vi "示波器主程序.vi"() -> ()   [LabVIEW 2018]
panel:
  in  "VISA资源名称":refnum<visa-resource-name>
  in  "要打开的通道":string[](array[string])
  out "波形图":u8[][](graph)
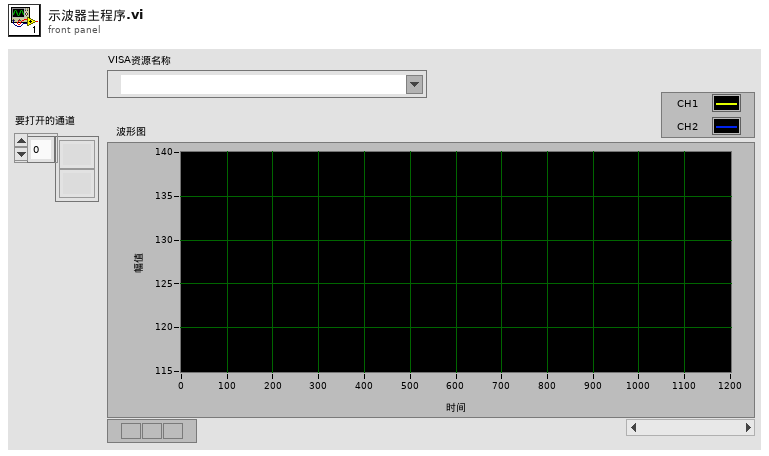
[diagram p1: front panel]
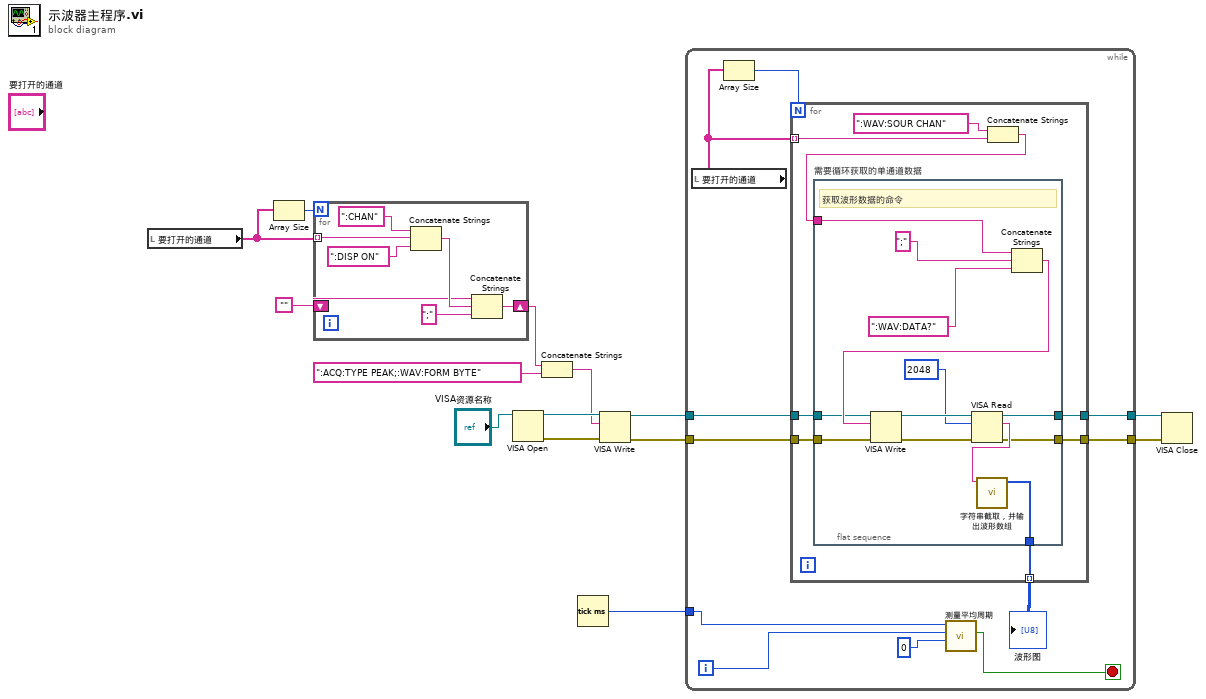
[diagram p0: block diagram]
diagram:
  n1 = local read "要打开的通道"() -> (w5:string[])
  n2 = Array Size(array=w5) -> (size(s)=w7:i32)
  n3 = for {
    N: w7 -> [_]
    tunnel: w5 -> [w21] mode=indexing
    shift-right: [w18] -> w3
    shift-left: "" -> [w16]
    n4 = Concatenate Strings(":CHAN" ("写入缓冲区"), w21, ":DISP ON" ("写入缓冲区")) -> (w17:string)
    n5 = Concatenate Strings(w16, w17, ";" ("写入缓冲区")) -> (w18:string)
  }
  n6 = VISA Open(VISA resource name="VISA资源名称") -> (VISA resource name=w9:refnum<visa-resource-name>, error out=w8:errorcluster)  [unwired: 4 in]
  n7 = Concatenate Strings(w3, ":ACQ:TYPE PEAK;:WAV:FORM BYTE") -> (w2:string)
  n8 = Tick Count (ms)() -> (millisecond timer value=w14:u32)
  n9 = VISA Write(VISA resource name=w9, write buffer=w2, error in (no error)=w8) -> (VISA resource name out=w10:refnum<visa-resource-name>, error out=w11:errorcluster)  [unwired: 1 out]
  n10 = while {
    tunnel: w14 -> [w28]
    tunnel: [w25] -> w13
    tunnel: [w24] -> w12
    tunnel: w10 -> [w23]
    tunnel: w11 -> [w22]
    i -> [w27]
    stop <- w26 stop-if-true
    n11 = local read "要打开的通道"() -> (w31:string[])
    n12 = Array Size(array=w31) -> (size(s)=w32:i32)
    n13 = for {
      N: w32 -> [_]
      tunnel: w31 -> [w39] mode=indexing
      tunnel: [w37] -> w30 mode=indexing
      tunnel: [w36] -> w25
      tunnel: [w35] -> w24
      tunnel: w23 -> [w34]
      tunnel: w22 -> [w33]
      n14 = flat-sequence "需要循环获取的单通道数据" {
        tunnel: w38 -> [w49]
        tunnel: [w47] -> w37
        tunnel: [w46] -> w36
        tunnel: [w45] -> w35
        tunnel: w34 -> [w42]
        tunnel: w33 -> [w41]
        frame #0 {
          # "获取波形数据的命令"
          n15 = Concatenate Strings(w49, ";" ("写入缓冲区"), ":WAV:DATA?" ("写入缓冲区")) -> (w50:string)
          n16 = VISA Write(VISA resource name=w42, write buffer=w50, error in (no error)=w41) -> (VISA resource name out=w53:refnum<visa-resource-name>, error out=w52:errorcluster)  [unwired: 1 out]
          n17 = VISA Read(VISA resource name=w53, byte count=u32 2048 ("字节总数"), error in (no error)=w52) -> (VISA resource name out=w46:refnum<visa-resource-name>, read buffer=w48:string, error out=w45:errorcluster)  [unwired: 1 out]
          n18 = call "字符串截取，并输出波形数组.vi"("read buffer"=w48) -> ("数组"=w47:u8[])  [unwired: 8 in, 2 out]
        }
      }
      n19 = Concatenate Strings(":WAV:SOUR CHAN" ("写入缓冲区"), w39) -> (w38:string)
    }
    "波形图" <- w30
    n20 = call "测量平均周期.vi"("运行总次数（为0则一直进行）"=u32 0 ("y"), "已运行次数（i+1）"=w27, "初始时间"=w28) -> ("布尔"=w26:bool)  [unwired: 7 in, 1 out]
  }
  n21 = VISA Close(VISA resource name=w13, error in (no error)=w12) -> ()  [unwired: 1 out]
